vi "getVIPath.vi"(8 "error in":errorcluster, 10 "Cluster in":T1, 11 "path":path) -> (0 "error out":errorcluster, 3 "Cluster out":T1)   [LabVIEW 2020]
doc: "Get stripped path from given VI"
uses:
  controls/StateMachineVariables.ctl
  <vilib>/vision/Avi.llb/IMAQ AVI2 Refnum.ctl
  <vilib>/userDefined/High Color/IMAQdx.ctl
  <vilib>/vision/Deep Learning.llb/IMAQ DL Model Refnum.ctl
  <vilib>/vision/Image Controls.llb/IMAQ Image.ctl
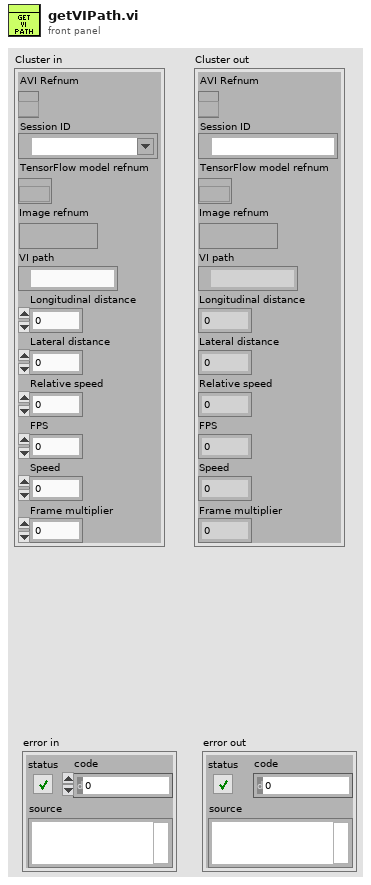
[diagram p1: front panel]
types:
  T1 = typedef "StateMachineVariables.ctl" = cluster{"AVI Refnum":T2, "Session ID":T3, "TensorFlow model refnum":T4, "Image refnum":T5, "VI path":path, "Longitudinal distance":dbl, "Lateral distance":dbl, "Relative speed":dbl, "FPS":dbl, "Speed":dbl, "Frame multiplier":u32}
  T2 = typedef "IMAQ AVI2 Refnum.ctl" = refnum<k20>
  T3 = typedef "IMAQdx.ctl" = refnum<k21>
  T4 = typedef "IMAQ DL Model Refnum.ctl" = refnum<k20>
  T5 = typedef "IMAQ Image.ctl" = refnum<image>
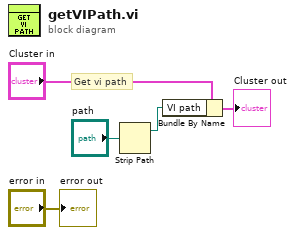
[diagram p0: block diagram]
diagram:
  # "Get vi path"
  n1 = Strip Path(path="path") -> (stripped path=w4:path)  [unwired: 1 out]
  n2 = Bundle By Name(cluster="Cluster in", "VI path"=w4) -> (→"Cluster out":T1)
  "error out" <- "error in"
